vi "Reinitialize.vi"(8 "error in (no error)":errorcluster, 11 "SOL MS in":refnum<class "PL SOL Instruments Camera.lvclass">) -> (0 "error out":errorcluster, 3 "SOL Camera out":refnum<class "PL SOL Instruments Camera.lvclass">)   [LabVIEW 2015, in "PL SOL Instruments Camera.lvclass"]
doc: "Reinitializes connection to device based on previously specified settings."
uses:
  PL SOL Instruments Camera.lvclass
  PL SOL Instruments Camera.lvclass/PL SOL Instruments Camera.ctl
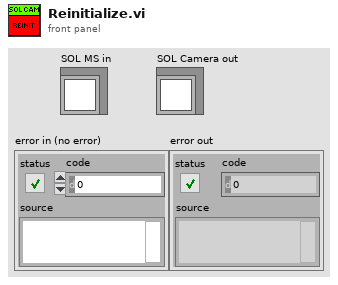
[diagram p1: front panel]
types:
  T1 = cluster{"wMaxHBinning":u16, "wMaxVBinning":u16, "wRegionsCount":u16, "wRegionsFlags":u16, "wMinRegionWidth":u16, "wMaxRegionWidth":u16, "wMinRegionHeight":u16, "wMaxRegionHeight":u16, "wFanCount":u16, "wSynchOutCount":u16, "wSynchModesCount":u16, "wSynchOut1ModesCount":u16, "wSynchOut2ModesCount":u16, "wCameraRAMSize":u16, "dwImagesToStore":u32}
  T2 = cluster{"wWidth":u16, "wHeight":u16, "wReadoutSpeedCount":u16, "wCoolingType":u16, "lTempMin":i32, "lTempMax":i32}
  T3 = cluster{"lOSMemory":i32, "dwOSMajorVer":u32, "dwOSMinorVer":u32, "dwOSPlatform":u32, "wSoftMajorVer":u16, "wSoftMinorVer":u16, "wFPGAMajorVer":u16, "wFPGAMinorVer":u16}
  T4 = cluster{"wMinRegionWidth":u16, "wMaxRegionWidth":u16}
  T5 = cluster{"wMinRegionHeight":u16, "wMaxRegionHeight":u16}
  T6 = cluster{bool, bool, bool, bool, bool, cluster{"wMinRegionWidth":u16, "wMaxRegionWidth":u16}, cluster{"wMinRegionHeight":u16, "wMaxRegionHeight":u16}}
  T7 = cluster{"memory size, MB":i32, "os":string, "software version":string, "FPGA version":string, "device name":string, "serial number":string}
  T8 = cluster{"frame":cluster{"width":u16, "height":u16}, "cooling":cluster{"type":u16, "temperature range":cluster{"min":i32, "max":i32}}, "readout rates, kHz":i32[], "pixel":cluster{"width, mkm":dbl, "height. mkm":dbl}, "max binning":cluster{"horizontal":u16, "vertical":u16}, "max number of regions":u16, "region size constraints":cluster{"even start":bool, "div by 4":bool, "div by 8":bool, "div by 16":bool, "fvb only":bool, "width":cluster{"min":u16, "max":u16}, "height":cluster{"min":u16, "max":u16}}, "number of fans":u16, "RAM":cluster{"size, MB":u16, "max number of frames":u32}, "number of outputs":u16, "number of synchronization modes":u16, "number of OUT1 modes":u16, "number of OUT2 modes":u16, "exposure time":cluster{"min, us":dbl, "max, s":dbl}, "delay before exposure":cluster{"min, s":dbl, "max, s":dbl}, "delay after exposure":cluster{"min, s":dbl, "max, s":dbl}, "delay between exposures":cluster{"min, s":dbl, "max, s":dbl}, "sensor type":u16}
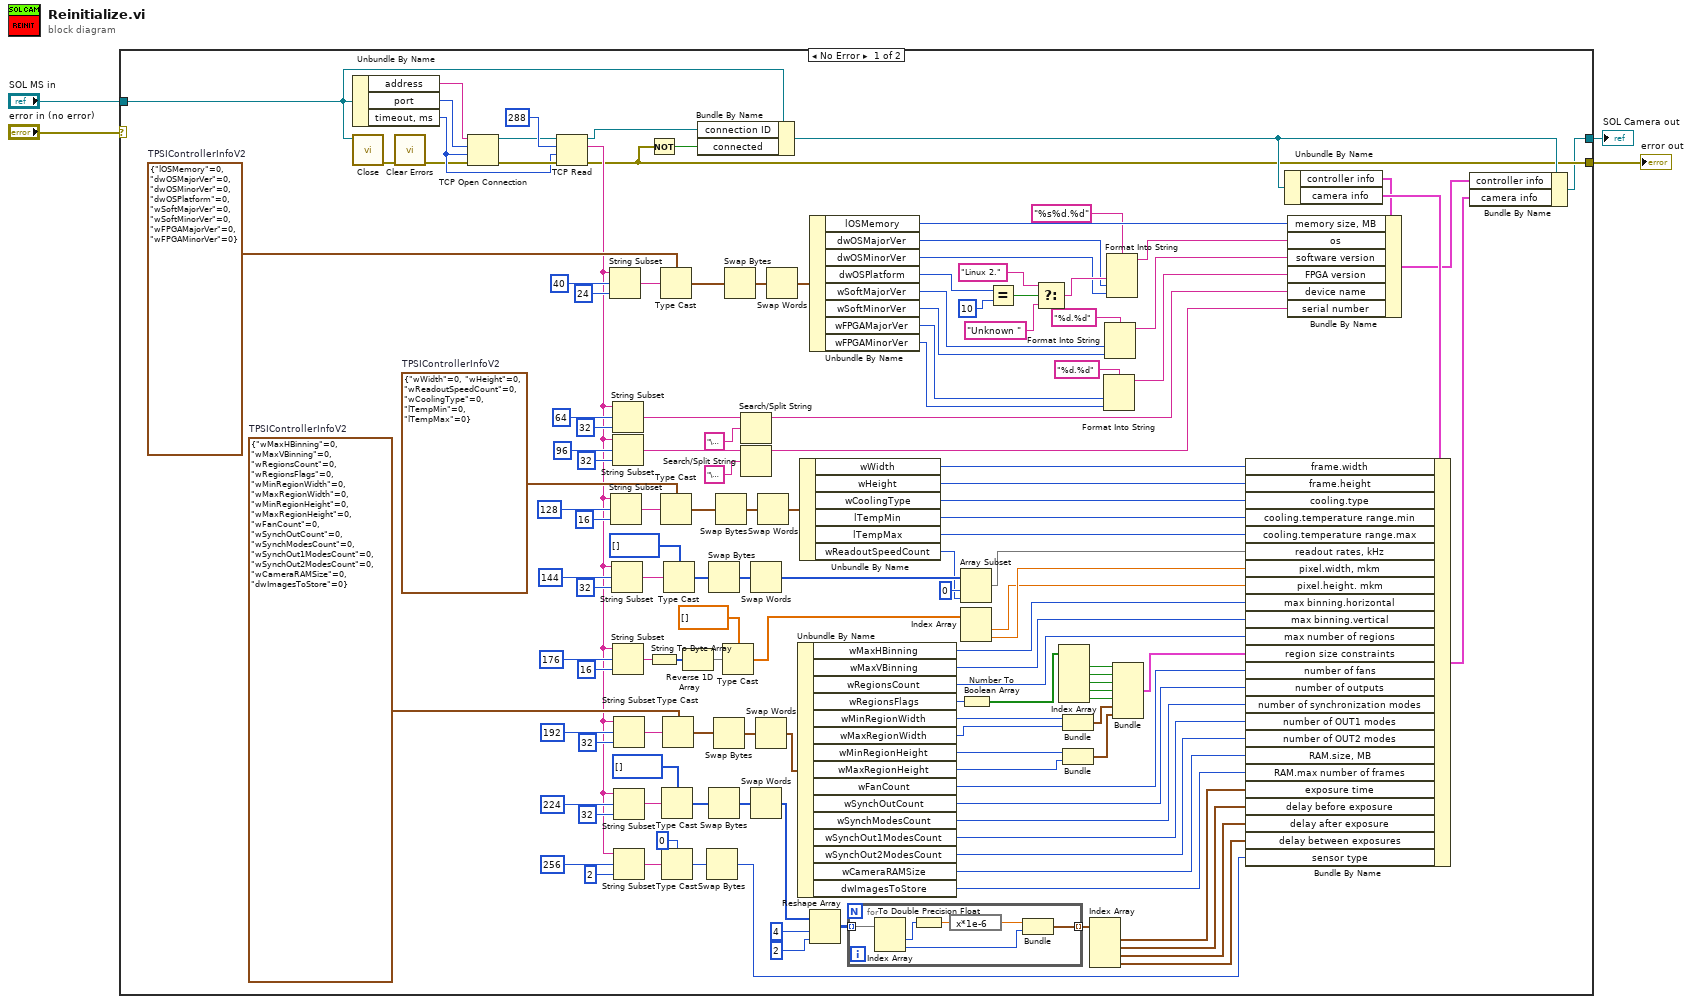
[diagram p0: block diagram]
diagram:
  n1 = case shown="No Error" "error in (no error)" {
    selector: "error in (no error)" -> [_ w149]
    tunnel: [w9 w149] -> w4
    tunnel: [w8 w150] -> w3
    tunnel: "SOL MS in" -> [w7 w150]
    frame No Error {
      w56 = T1 {"wMaxHBinning"=0, "wMaxVBinning"=0, "wRegionsCount"=0, "wRegionsFlags"=0, "wMinRegionWidth"=0, "wMaxRegionWidth"=0, "wMinRegionHeight"=0, "wMaxRegionHeight"=0, "wFanCount"=0, "wSynchOutCount"=0, "wSynchModesCount"=0, "wSynchOut1ModesCount"=0, "wSynchOut2ModesCount"=0, "wCameraRAMSize"=0, "dwImagesToStore"=0}  # TPSIControllerInfoV2
      w100 = T2 {"wWidth"=0, "wHeight"=0, "wReadoutSpeedCount"=0, "wCoolingType"=0, "lTempMin"=0, "lTempMax"=0}  # TPSIControllerInfoV2
      w130 = T3 {"lOSMemory"=0, "dwOSMajorVer"=0, "dwOSMinorVer"=0, "dwOSPlatform"=0, "wSoftMajorVer"=0, "wSoftMinorVer"=0, "wFPGAMajorVer"=0, "wFPGAMinorVer"=0}  # TPSIControllerInfoV2
      n2 = Unbundle By Name(w7) -> ("address"=w11:string, "port"=w10:u16, "timeout, ms"=w12:u32)
      n3 = call "Close.vi"("SOL Camera in"=w7) -> ("error out"=w6:errorcluster)  [unwired: 10 in]
      n4 = call <vilib>:"Clear Errors.vi"("error in (no error)"=w6) -> ("error out"=w5:errorcluster)  [unwired: 5 in, 1 out]
      n5 = TCP Open Connection(address=w11, remote port or service name=w10, timeout ms (60000)=w12, error in (no error)=w5) -> (connection ID=w19:refnum<k5>, error out=w18:errorcluster)  [unwired: 1 in]
      n6 = TCP Read(connection ID=w19, bytes to read=288, error in (no error)=w18, 9:w12) -> (connection ID out=w17:refnum<k5>, data out=w28:string, error out=w9:errorcluster)  [unwired: 1 in]
      n7 = String Subset(string=w28, offset (0)=40, length (rest)=24 ("length (rest)")) -> (substring=w131:string)
      n8 = String Subset(string=w28, offset (0)=128, length (rest)=16 ("length (rest)")) -> (substring=w101:string)
      n9 = String Subset(string=w28, offset (0)=144, length (rest)=32 ("length (rest)")) -> (substring=w85:string)
      n10 = String Subset(string=w28, offset (0)=64, length (rest)=32 ("length (rest)")) -> (substring=w107:string)
      n11 = String Subset(string=w28, offset (0)=96, length (rest)=32 ("length (rest)")) -> (substring=w106:string)
      n12 = String Subset(string=w28, offset (0)=176, length (rest)=16 ("length (rest)")) -> (substring=w52:string)
      n13 = String Subset(string=w28, offset (0)=192, length (rest)=32 ("length (rest)")) -> (substring=w59:string)
      n14 = String Subset(string=w28, offset (0)=224, length (rest)=32 ("length (rest)")) -> (substring=w42:string)
      n15 = String Subset(string=w28, offset (0)=256, length (rest)=2 ("length (rest)")) -> (substring=w27:string)
      n16 = Not(x=w9) -> (.not. x?=w16:bool)
      n17 = String To Byte Array(string=w52) -> (unsigned byte array=w51:u8[])
      n18 = Type Cast(type=w130, x=w131) -> (*(type *) &x=w129:T3)
      n19 = Type Cast(type=w100, x=w101) -> (*(type *) &x=w98:T2)
      n20 = Type Cast(type=u32[] [], x=w42) -> (*(type *) &x=w40:u32[])
      n21 = Type Cast(type=u16 0, x=w27) -> (*(type *) &x=w25:u16)
      n22 = Type Cast(type=w56, x=w59) -> (*(type *) &x=w55:T1)
      n23 = Type Cast(type=i32[] [], x=w85) -> (*(type *) &x=w84:i32[])
      n24 = Reverse 1D Array(array=w51) -> (reversed array=w48:u8[])
      n25 = Bundle By Name(cluster=w7, "connection ID"=w17, "connected"=w16) -> (w13:refnum<class "PL SOL Instruments Camera.lvclass">)
      n26 = Swap Bytes(anything=w25) -> (byte swapped=w24:u16)
      n27 = Swap Bytes(anything=w84) -> (byte swapped=w92:i32[])
      n28 = Swap Bytes(anything=w40) -> (byte swapped=w41:u32[])
      n29 = Swap Bytes(anything=w55) -> (byte swapped=w54:T1)
      n30 = Swap Bytes(anything=w98) -> (byte swapped=w99:T2)
      n31 = Type Cast(type=dbl[] [], x=w48) -> (*(type *) &x=w49:dbl[])
      n32 = Swap Bytes(anything=w129) -> (byte swapped=w105:T3)
      n33 = Search/Split String(string=w107, search string/char (-)="\u0000") -> (substring before match=w109:string)  [unwired: 1 in, 2 out]
      n34 = Search/Split String(string=w106, search string/char (-)="\u0000") -> (substring before match=w108:string)  [unwired: 1 in, 2 out]
      n35 = Swap Words(1:w92) -> (0:w91:i32[])
      n36 = Swap Words(1:w41) -> (0:w39:u32[])
      n37 = Swap Words(1:w54) -> (0:w53:T1)
      n38 = Swap Words(1:w99) -> (0:w97:T2)
      n39 = Swap Words(1:w105) -> (0:w104:T3)
      n40 = Unbundle By Name(w53) -> ("wMaxHBinning"=w83:u16, "wMaxVBinning"=w82:u16, "wRegionsCount"=w81:u16, "wRegionsFlags"=w80:u16, "wMinRegionWidth"=w73:u16, "wMaxRegionWidth"=w72:u16, "wMinRegionHeight"=w71:u16, "wMaxRegionHeight"=w70:u16, "wFanCount"=w66:u16, "wSynchOutCount"=w65:u16, "wSynchModesCount"=w64:u16, "wSynchOut1ModesCount"=w63:u16, "wSynchOut2ModesCount"=w62:u16, "wCameraRAMSize"=w61:u16, "dwImagesToStore"=w60:u32)
      n41 = Unbundle By Name(w97) -> ("wWidth"=w15:u16, "wHeight"=w14:u16, "wCoolingType"=w96:u16, "lTempMin"=w95:i32, "lTempMax"=w94:i32, "wReadoutSpeedCount"=w89:u16)
      n42 = Unbundle By Name(w104) -> ("lOSMemory"=w128:i32, "dwOSMajorVer"=w117:u32, "dwOSMinorVer"=w116:u32, "dwOSPlatform"=w126:u32, "wSoftMajorVer"=w115:u16, "wSoftMinorVer"=w114:u16, "wFPGAMajorVer"=w113:u16, "wFPGAMinorVer"=w112:u16)
      n43 = Reshape Array(w39, 4 ("dimension size"), 2 ("dimension size")) -> (w36:u32[][])
      n44 = for {
        tunnel: w36 -> [w148] mode=indexing
        tunnel: [w145] -> w35 mode=indexing
        n45 = Index Array(array=w148) -> (element #1=w147:u32, element #2=w143:u32)  [unwired: 2 in]
        n46 = To Double Precision Float(number=w147) -> (double precision float=w146:dbl)
        n47 = expression code="x*1e-6"(w146) -> (w144:dbl)
        n48 = Bundle(w144, w143) -> (w145:cluster{dbl, u32})  [unwired: 1 in]
      }
      n49 = Array Subset(array=w91, index=0, length=w89) -> (w88:i32[])
      n50 = Index Array(array=w49) -> (element #1=w46:dbl, element #2=w47:dbl)  [unwired: 2 in]
      n51 = Number To Boolean Array(number=w80) -> (Boolean array=w79:bool[])
      n52 = Equal?(x=w126, y=u32 10) -> (x = y?=w124:bool)
      n53 = Select(t="Linux 2." ("format string"), s=w124, f="Unknown " ("format string")) -> (s? t:f=w121:string)
      n54 = Index Array(array=w79) -> (element #1=w78:bool, element #2=w74:bool, element #3=w75:bool, element #4=w76:bool, element #5=w77:bool)  [unwired: 5 in]
      n55 = Bundle("wMinRegionWidth"=w73, "wMaxRegionWidth"=w72) -> (w68:T4)  [unwired: 1 in]
      n56 = Bundle("wMinRegionHeight"=w71, "wMaxRegionHeight"=w70) -> (w69:T5)  [unwired: 1 in]
      n57 = Index Array(array=w35) -> (element #1=w34:cluster{dbl, u32}, element #2=w33:cluster{dbl, u32}, element #3=w32:cluster{dbl, u32}, element #4=w31:cluster{dbl, u32})  [unwired: 4 in]
      n58 = Format Into String(format string="%d.%d", w113, w112) -> (resulting string=w110:string)  [unwired: 2 in, 1 out]
      n59 = Format Into String(format string="%d.%d", w115, w114) -> (resulting string=w111:string)  [unwired: 2 in, 1 out]
      n60 = Format Into String(format string="%s%d.%d", w121, w117, w116) -> (resulting string=w120:string)  [unwired: 2 in, 1 out]
      n61 = Bundle(w78, w74, w75, w76, w77, w68, w69) -> (w67:T6)  [unwired: 1 in]
      n62 = Unbundle By Name(w13) -> ("controller info"=w21:T7, "camera info"=w23:T8)
      n63 = Bundle By Name(cluster=w23, "frame.width"=w15, "frame.height"=w14, "cooling.type"=w96, "cooling.temperature range.min"=w95, "cooling.temperature range.max"=w94, "readout rates, kHz"=w88, "pixel.width, mkm"=w47, "pixel.height. mkm"=w46, "max binning.horizontal"=w83, "max binning.vertical"=w82, "max number of regions"=w81, "region size constraints"=w67, "number of fans"=w66, "number of outputs"=w65, "number of synchronization modes"=w64, "number of OUT1 modes"=w63, "number of OUT2 modes"=w62, "RAM.size, MB"=w61, "RAM.max number of frames"=w60, "exposure time"=w34, "delay before exposure"=w33, "delay after exposure"=w32, "delay between exposures"=w31, "sensor type"=w24) -> (w22:T8)
      n64 = Bundle By Name(cluster=w21, "memory size, MB"=w128, "os"=w120, "software version"=w111, "FPGA version"=w110, "device name"=w109, "serial number"=w108) -> (w20:T7)
      n65 = Bundle By Name(cluster=w13, "controller info"=w20, "camera info"=w22) -> (w8:refnum<class "PL SOL Instruments Camera.lvclass">)
    }
    frame Error {
    }
  }
  "SOL Camera out" <- w3
  "error out" <- w4
